vi "Main.vi"() -> (0 "error out":errorcluster)   [LabVIEW 2017, in "Sound Demo.lvclass"]
doc: "This is the top-level VI that starts the Sound Player Demo application."
uses:
  Sound Demo.lvclass
  C:/GitRepos/SoundDemoProject/Application/Application.lvclass
  Application/Application.lvclass
panel:
  out "number (0 to 1)":dbl
  # "This is the top-level VI of the \nSound Player Demo project."
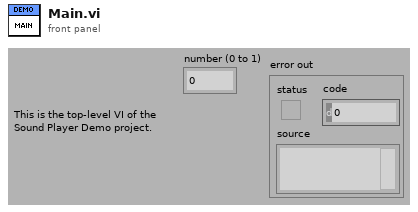
[diagram p1: front panel]
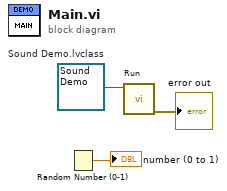
[diagram p0: block diagram]
diagram:
  w2 = refnum<class "Sound Demo.lvclass"> refnum  # Sound Demo.lvclass
  n1 = Random Number (0-1)() -> (number: 0 to 1=→"number (0 to 1)":dbl)
  n2 = call "Run.vi"("Application in"=w2) -> ("error out"=→"error out":errorcluster)  [unwired: 9 in, 1 out]
